vi "RX MEI Data.vi"(8 "error in (no error)":errorcluster, 11 "VISA resource in":refnum<visa-resource-name>) -> (0 "error out":errorcluster, 1 "CRC":string, 2 "Data Buffer":string, 3 "VISA resource out":refnum<visa-resource-name>)   [LabVIEW 2012, in "MB Master.lvlib" / "MB_ADU_RTU.lvclass"]
uses:
  MB_ADU_RTU.lvclass
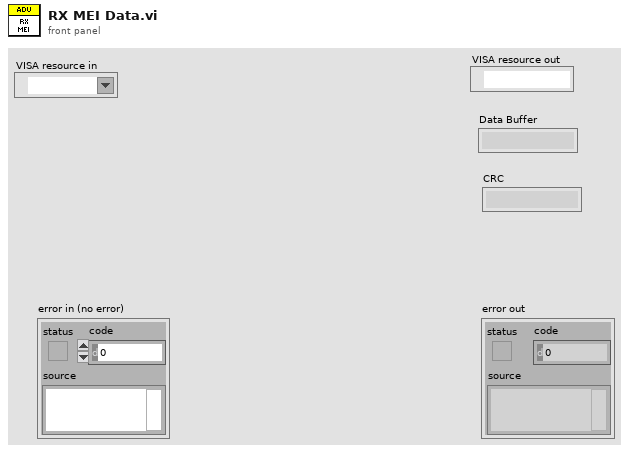
[diagram p1: front panel]
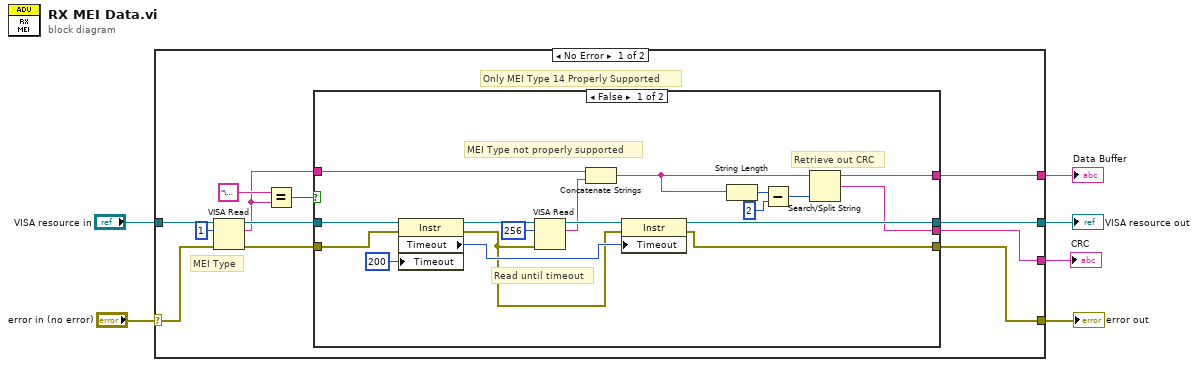
[diagram p0: block diagram]
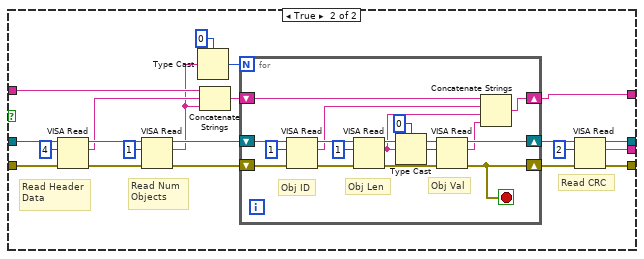
[diagram p2: hidden frame]
diagram:
  n1 = case shown="No Error" "error in (no error)" {
    selector: "error in (no error)" -> [w17 w76]
    tunnel: [w9 w76] -> w5
    tunnel: "VISA resource in" -> [w16 w75]
    tunnel: [w8 _] -> w3
    tunnel: [w10 w75] -> w2
    tunnel: [w7 _] -> w1
    frame No Error {
      # "Only MEI Type 14 Properly Supported"
      # "MEI Type"
      n2 = VISA Read(VISA resource name=w16, byte count=u32 1, error in (no error)=w17) -> (VISA resource name out=w15:refnum<visa-resource-name>, read buffer=w11:string, error out=w12:errorcluster)  [unwired: 1 out]
      n3 = Equal?(x="\u000e", y=w11) -> (x = y?=w13:bool)
      n4 = case shown="False" w13 {
        tunnel: w15 -> [w35 w55]
        tunnel: w12 -> [w33 w56]
        tunnel: w11 -> [w29 w47]
        tunnel: [w20 w43] -> w8
        tunnel: [w26 w40] -> w10
        tunnel: [w27 w39] -> w9
        tunnel: [w19 w37] -> w7
        frame False {
          # "Retrieve out CRC"
          # "MEI Type not properly supported"
          # "Read until timeout"
          n5 = property class="Instr"(reference=w35, error in=w33, "Timeout"=u32 200 ("General Settings:Timeout Value")) -> (reference out=w32:refnum<visa-resource-name>, error out=w25:errorcluster, "Timeout"=w30:u32)
          n6 = VISA Read(VISA resource name=w32, byte count=u32 256, error in (no error)=w25) -> (VISA resource name out=w31:refnum<visa-resource-name>, read buffer=w28:string)  [unwired: 2 out]
          n7 = Concatenate Strings(w29, w28) -> (w21:string)
          n8 = property class="Instr"(reference=w31, error in=w25, "Timeout"=w30) -> (reference out=w26:refnum<visa-resource-name>, error out=w27:errorcluster)
          n9 = String Length(string=w21) -> (length=w23:i32)
          n10 = Subtract(x=w23, y=2) -> (x-y=w22:i32)
          n11 = Search/Split String(string=w21, offset (0)=w22) -> (substring before match=w20:string, match + rest of string=w19:string)  [unwired: 1 in, 1 out]
        }
        frame True {
          # "Read CRC"
          # "Read Num\nObjects"
          # "Read Header\nData"
          n12 = VISA Read(VISA resource name=w55, byte count=u32 4, error in (no error)=w56) -> (VISA resource name out=w53:refnum<visa-resource-name>, read buffer=w46:string, error out=w52:errorcluster)  [unwired: 1 out]
          n13 = VISA Read(VISA resource name=w53, byte count=u32 1, error in (no error)=w52) -> (VISA resource name out=w49:refnum<visa-resource-name>, read buffer=w45:string, error out=w48:errorcluster)  [unwired: 1 out]
          n14 = Type Cast(type=u8 0, x=w45) -> (*(type *) &x=w50:u8)
          n15 = Concatenate Strings(w47, w46, w45) -> (w44:string)
          n16 = for {
            N: w50 -> [_]
            shift-right: [w63] -> w38
            shift-left: w48 -> [w73]
            shift-right: [w64] -> w41
            shift-left: w49 -> [w74]
            shift-right: [w61] -> w43
            shift-left: w44 -> [w60]
            stop <- w63 stop-if-true
            # "Obj Val"
            # "Obj Len"
            # "Obj ID"
            n17 = VISA Read(VISA resource name=w74, byte count=u32 1, error in (no error)=w73) -> (VISA resource name out=w71:refnum<visa-resource-name>, read buffer=w59:string, error out=w69:errorcluster)  [unwired: 1 out]
            n18 = VISA Read(VISA resource name=w71, byte count=u32 1, error in (no error)=w69) -> (VISA resource name out=w66:refnum<visa-resource-name>, read buffer=w58:string, error out=w65:errorcluster)  [unwired: 1 out]
            n19 = Type Cast(type=u8 0, x=w58) -> (*(type *) &x=w67:u8)
            n20 = VISA Read(VISA resource name=w66, byte count=w67, error in (no error)=w65) -> (VISA resource name out=w64:refnum<visa-resource-name>, read buffer=w62:string, error out=w63:errorcluster)  [unwired: 1 out]
            n21 = Concatenate Strings(w60, w59, w58, w62) -> (w61:string)
          }
          n22 = VISA Read(VISA resource name=w41, byte count=u32 2, error in (no error)=w38) -> (VISA resource name out=w40:refnum<visa-resource-name>, read buffer=w37:string, error out=w39:errorcluster)  [unwired: 1 out]
        }
      }
    }
    frame Error {
    }
  }
  "error out" <- w5
  "VISA resource out" <- w2
  "Data Buffer" <- w3
  "CRC" <- w1
